vi "Wait for Target Gallons.vi"(0 ".NET Refnum in":refnum<k24>, 5 "GEA Inputs":T1 {"Destination" format="%.0x"; "Source" format="%.0x"}, 9 "Target Gallons":dbl, 11 "error in (no error)":errorcluster) -> (4 "GEA2 Reference Out":refnum<k24>, 15 "error out":errorcluster)   [LabVIEW 2018, in "TLMB.lvlib"]
uses:
  Projects/TLMB.lvlib
  D:/Common/LabVIEW GEA2 Toolkit/source/GEA3 DLL Source/GeaCommunication.dll
  Common/LabVIEW GEA2 Toolkit/source/GEA3 DLL Source/GeaCommunication.dll
  Common/LabVIEW GEA2 Toolkit/GEA3/type defs/Source_Destination.ctl
  Common/LabVIEW GEA2 Toolkit/GEA3/type defs/ERD Read Data In.ctl
  Common/LabVIEW GEA2 Toolkit/GEA3/type defs/Data Type.ctl
  C:/Users/iallatyp/Desktop/New folder/GEA3/library/GEA2_Toolkit.lvlib
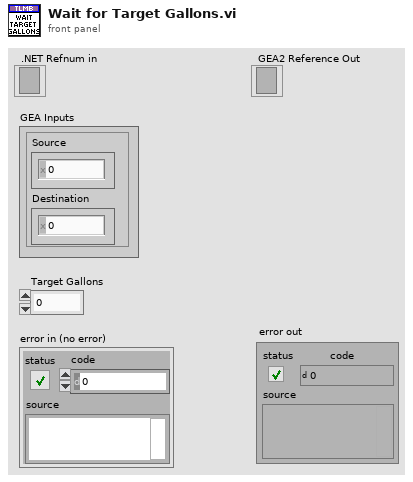
[diagram p1: front panel]
types:
  T1 = typedef "GEA2_Toolkit.lvlib/Source_Destination.ctl" = cluster{"Source":u8, "Destination":u8}
  T2 = typedef "GEA2_Toolkit.lvlib/ERD Read Data In.ctl" = cluster{"ERD Number":u16, "Data Type":T3}
  T3 = typedef "GEA2_Toolkit.lvlib/Data Type.ctl" = enum16{"string", "boolean", "uint8_t", "uint16_t", "uint32_t", "uint64_t", "int8_t", "int16_t", "int32_t", "int64_t"}
  T4 = typedef "GEA2_Toolkit.lvlib/ERD Read Data Out.ctl" = cluster{"ERD Number":u16, "Data":string}
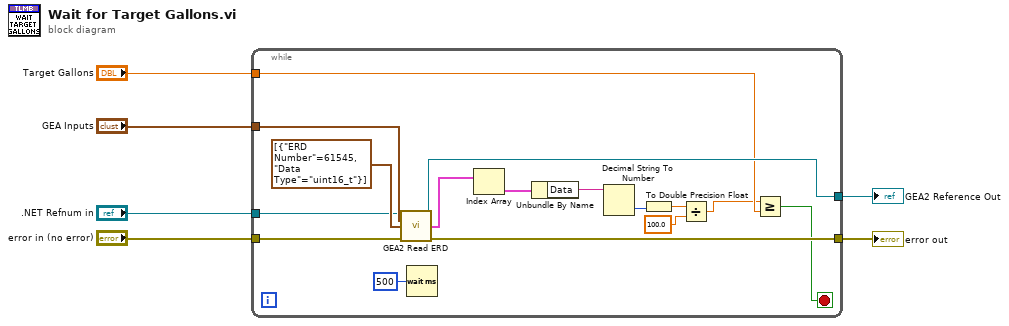
[diagram p0: block diagram]
diagram:
  n1 = while {
    tunnel: "error in (no error)" -> [w21]
    tunnel: [w20] -> w2
    tunnel: "GEA Inputs" -> [w19]
    tunnel: ".NET Refnum in" -> [w18]
    tunnel: "Target Gallons" -> [w9]
    tunnel: [w10] -> w1
    stop <- w11 stop-if-true
    n2 = call "GEA2 Read ERD.vi"("GEA2 Reference In"=w18, "GEA Inputs"=w19, "Read ERD List"=T2[] [{"ERD Number"=61545, "Data Type"=enum."uint16_t"}], "Error In"=w21) -> ("GEA2 Reference Out"=w10:refnum<k24>, "ERD Data Out"=w17:T4[], "Error Out"=w20:errorcluster)  [unwired: 8 in, 1 out]
    n3 = Wait (ms)(milliseconds to wait=u32 500) -> ()  [unwired: 1 out]
    n4 = Index Array(array=w17) -> (element=w16:T4)  [unwired: 1 in]
    n5 = Unbundle By Name(w16) -> ("Data"=w15:string)
    n6 = Decimal String To Number(string=w15) -> (number=w14:i32)  [unwired: 2 in, 1 out]
    n7 = To Double Precision Float(number=w14) -> (double precision float=w13:dbl)
    n8 = Divide(x=w13, y=100.0) -> (x/y=w8:dbl)
    n9 = Greater Or Equal?(x=w8, y=w9) -> (x >= y?=w11:bool)
  }
  "error out" <- w2
  "GEA2 Reference Out" <- w1
